vi "Close.vi"(8 "error in":errorcluster, 9 "timeout (-1)":i32=-1, 11 "Standard Engine in":refnum<class "Standard Engine Runtime.lvclass">) -> (0 "error out":errorcluster)   [LabVIEW 2013, in "Standard Engine Runtime.lvclass"]
doc: "This VI halts the execution of the engine background process and closes any references to it. The 'Stop' method should be called first so that the engine background process has a chance to properly uninitialize itself."
uses:
  Standard Engine Runtime.lvclass
  <vilib>/NI/Module Execution Interface/Engine Runtime/Execution States.ctl
  Standard Engine Runtime.lvclass/Standard Engine Runtime.ctl
  Commands.ctl
  <vilib>/NI/Module Execution Interface/Engine Runtime/Engine Runtime Interface.lvclass
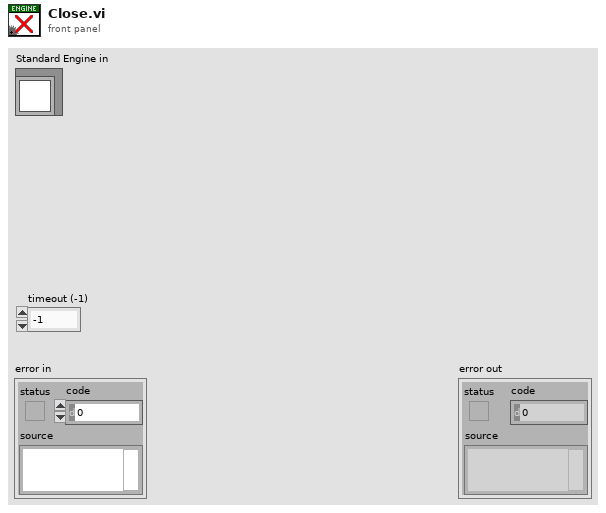
[diagram p1: front panel]
types:
  T1 = typedef "Engine Runtime Interface.lvclass/Execution States.ctl" = enum16{"Initializing", "Paused (Initialized)", "Running", "Set Safe Outputs", "Uninitializing", "Stopped (Uninitialized)", "Error (Uninitialized)", "Safe State (Uninitialized)", "Closed"}
  T2 = typedef "Standard Engine Runtime.lvclass/Commands.ctl" = enum16{"Initialize", "Start", "Pause", "Safe State", "Normal", "Stop", "Shutdown"}
  T3 = enum32{"Bad", "Idle", "Run top level", "Running"}
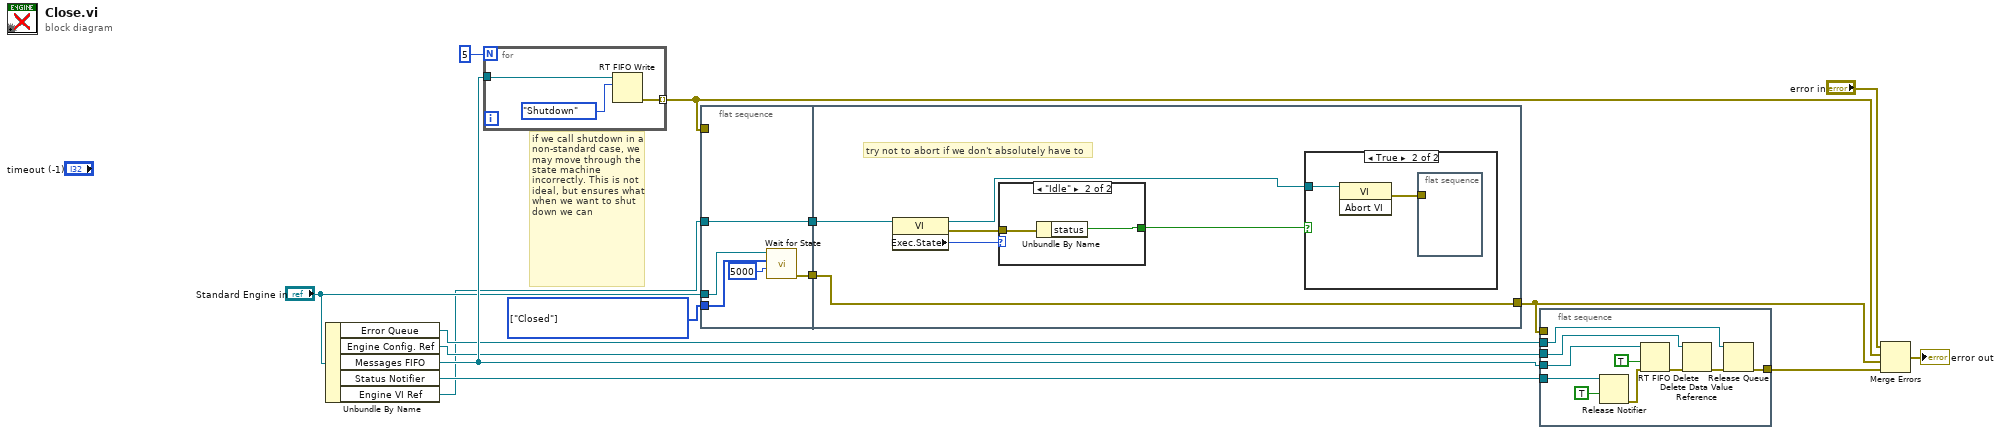
[diagram p0: block diagram]
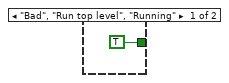
[diagram p2: hidden frame]
diagram:
  w13 = T1[] [enum."Closed"] items=["Initializing", "Paused (Initialized)", "Running", "Set Safe Outputs", "Uninitializing", "Stopped (Uninitialized)", "Error (Uninitialized)", "Safe State (Uninitialized)", "Closed"] ("expected states")
  # "if we call shutdown in a non-standard case, we may move through the state machine incorrectly. This is not ideal, but ensures what when we want to shut down we can"
  n1 = Unbundle By Name("Standard Engine in") -> ("Error Queue"=w7:refnum<queue>, "Engine Config. Ref"=w14:refnum<data-value>, "Messages FIFO"=w15:refnum<k33>, "Status Notifier"=w12:refnum<notifier>, "Engine VI Ref"=w3:refnum<vi>)
  n2 = for {
    N: 5 -> [_]
    tunnel: w15 -> [w16]
    tunnel: [w17] -> w5 mode=indexing
    n3 = RT FIFO Write(0:w16, 1:Commands."Shutdown" ("element")) -> (11:w17:errorcluster)  [unwired: 3 in, 3 out]
  }
  n4 = flat-sequence {
    tunnel: w13 -> [w22]
    tunnel: "Standard Engine in" -> [w21]
    tunnel: w5 -> [_]
    tunnel: [w20] -> w4
    tunnel: w3 -> [w20]
    tunnel: [w19] -> w2
    tunnel: w4 -> [w28]
    tunnel: w2 -> [w29]
    tunnel: [w29] -> w1
    frame #0 {
      n5 = call "Wait for State.vi"("timeout in ms"=5000, "expected states"=w22, "Standard Engine in"=w21) -> ("error out"=w19:errorcluster)  [unwired: 7 in, 1 out]
    }
    frame #1 {
      # "try not to abort if we don't absolutely have to"
      n6 = property class="VI"(reference=w28) -> (reference out=w26:refnum<vi>, error out=w24:errorcluster, "Exec.State"=w25:T3)  [unwired: 1 in]
      n7 = case shown="\"Idle\"" w25 {
        tunnel: w24 -> [_ w32]
        tunnel: [TRUE ("status") w31] -> w27
        frame "Bad", "Run top level", "Running" {
        }
        frame "Idle" {
          n8 = Unbundle By Name(w32) -> ("status"=w31:bool)
        }
      }
      n9 = case shown="True" w27 {
        tunnel: w26 -> [_ w34]
        frame False {
        }
        frame True {
          n10 = invoke class="VI" method="Abort VI"(reference=w34) -> (error out=w33:errorcluster)  [unwired: 2 in, 2 out]
          n11 = flat-sequence {
            tunnel: w33 -> [_]
            frame #0 {
            }
          }
        }
      }
    }
  }
  n12 = flat-sequence {
    tunnel: w15 -> [w44]
    tunnel: w14 -> [w41]
    tunnel: w12 -> [w39]
    tunnel: [w36] -> w8
    tunnel: w7 -> [w35]
    tunnel: w1 -> [_]
    frame #0 {
      n13 = Release Notifier(notifier=w39, force destroy? (F)=TRUE) -> (error out=w38:errorcluster)  [unwired: 1 in, 2 out]
      n14 = RT FIFO Delete(0:w44, 2:TRUE ("force destroy? (F)"), 3:w38) -> (11:w43:errorcluster)
      n15 = Delete Data Value Reference(data value reference=w41, error in=w43) -> (error out=w37:errorcluster)  [unwired: 1 out]
      n16 = Release Queue(queue=w35, error in (no error)=w37) -> (error out=w36:errorcluster)  [unwired: 1 in, 2 out]
    }
  }
  n17 = Merge Errors("error in", w5, w1, w8) -> (→"error out":errorcluster)
